vi "REQ Initialize Output.vi"(8 "error in (no error)":errorcluster, 9 "DAQ Type":enum16{"Hardware", "Simulation"}(ring), 10 "CAN Output":T1 {"data"."payload" format="%x"; "data"."timestamp" format="%<%.7X\n%x>T"; "data"."type" items=["CAN Data"=0, "CAN Remote"=1, "CAN Bus Error"=2, "CAN 2.0 Data"=8, "CAN FD Data"=16, "CAN FD+BRS Data"=24, "J1939 Data"=192, "Delay"=224, "Log Trigger"=225, "Start Trigger"=226]; "data"."identifier" format="%x"}, 11 "Abstract in":refnum<class "Abstract.lvclass">) -> (0 "error out":errorcluster, 3 "Abstract out":refnum<class "Abstract.lvclass">)   [LabVIEW 2021, in "CAN.lvlib" / "Abstract.lvclass"]
uses:
  Abstract.lvclass
  CAN Output.ctl
  <vilib>/xnet/xnet.llb/XNET Frame CAN.ctl
  <vilib>/xnet/xnet.llb/XNET Frame Type CAN.ctl
  CAN.lvlib
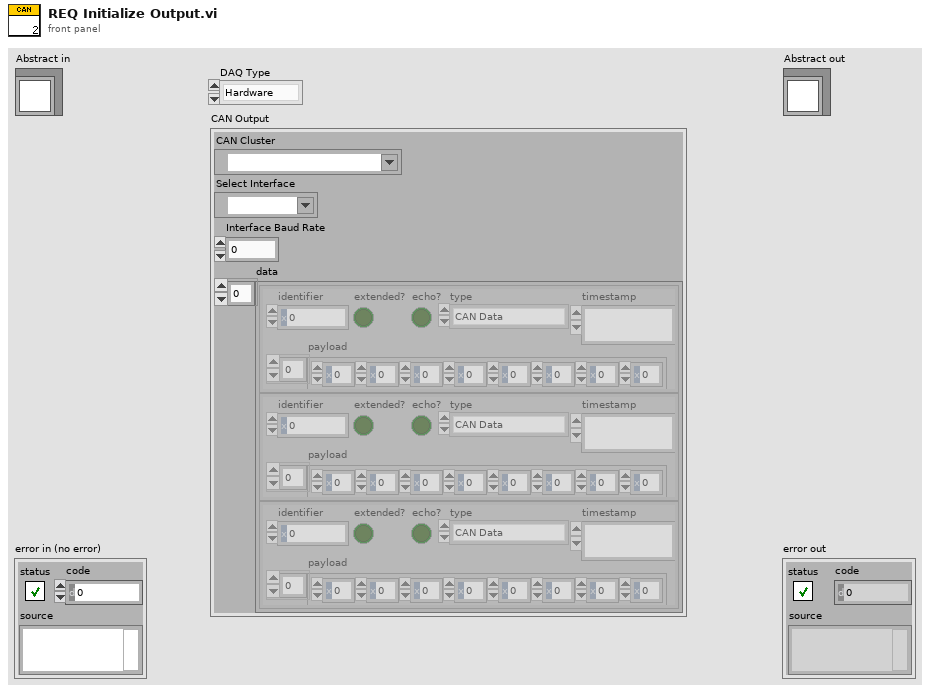
[diagram p1: front panel]
types:
  T1 = typedef "CAN.lvlib/CAN Output.ctl" = cluster{"CAN Cluster":refnum<k21>, "Select Interface":refnum<k21>, "Interface Baud Rate":u32, "data":T2[]}
  T2 = typedef "XNET Frame CAN.ctl" = cluster{"timestamp":timestamp, "payload":u8[], "identifier":u32, "type":T3, "extended?":bool, "echo?":bool}
  T3 = typedef "XNET Frame Type CAN.ctl" = u8
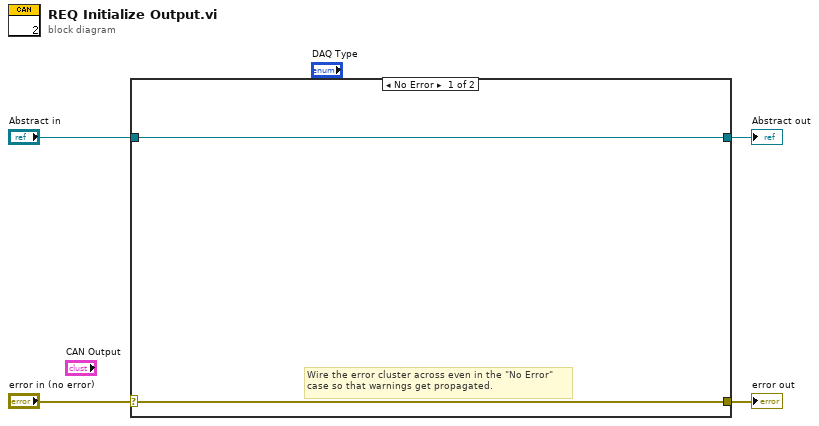
[diagram p0: block diagram]
diagram:
  n1 = case shown="No Error" "error in (no error)" {
    selector: "error in (no error)" -> [w5 w8]
    tunnel: [w5 w8] -> w3
    tunnel: [w6 w7] -> w1
    tunnel: "Abstract in" -> [w6 w7]
    frame No Error {
      # "Wire the error cluster across even in the \"No Error\"\ncase so that warnings get propagated."
    }
    frame Error {
    }
  }
  "error out" <- w3
  "Abstract out" <- w1
